vi "Set Arm (Bool).vi"(8 "error in (no error)":errorcluster, 10 "Down":bool, 11 "Up":bool) -> (0 "error out":errorcluster)   [LabVIEW 2011]
uses:
  Apendage State.ctl
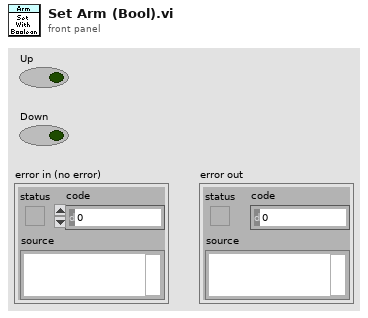
[diagram p1: front panel]
types:
  T1 = typedef "Apendage State.ctl" = enum16{"Unknown", "Down", "Up"}
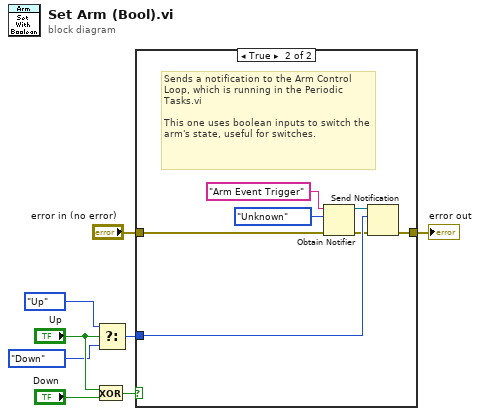
[diagram p0: block diagram]
diagram:
  n1 = Exclusive Or(1:"Down", 2:"Up") -> (0:w5:bool)
  n2 = Select(t=Apendage_State."Up", s="Up", f=Apendage_State."Down") -> (s? t:f=w6:T1)
  n3 = case shown="True" w5 {
    tunnel: w6 -> [_ w14]
    tunnel: "error in (no error)" -> [w9 w12]
    tunnel: [w9 w11] -> w8
    frame False {
    }
    frame True {
      # "Sends a notification to the Arm Control Loop, which is running in the Periodic Tasks.vi\n\nThis one uses boolean inputs to switch the arm's state, useful for switches."
      n4 = Obtain Notifier(name (unnamed)="Arm Event Trigger", notification data type=Apendage_State."Unknown", error in (no error)=w12) -> (notifier out=w15:refnum<notifier>, error out=w13:errorcluster)  [unwired: 1 in, 1 out]
      n5 = Send Notification(notification=w14, notifier=w15, error in (no error)=w13) -> (error out=w11:errorcluster)  [unwired: 1 out]
    }
  }
  "error out" <- w8
